vi "Check wether Click is in Plot Area.vi"(9 "Mouse Click Coordinates":T2, 11 "Plot Bounds":T1) -> (3 "Is in Plot Area?":bool)   [LabVIEW 2019]
uses:
  <vilib>/Utility/miscctls.llb/LVPoint32TypeDef.ctl
  <vilib>/Utility/miscctls.llb/LVRectTypeDef.ctl
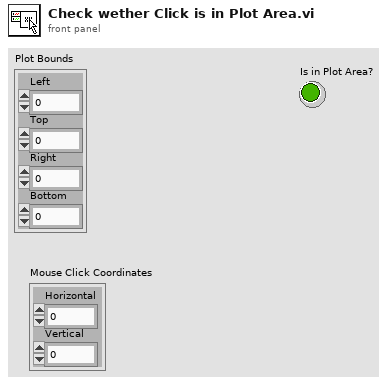
[diagram p1: front panel]
types:
  T1 = typedef "LVRectTypeDef.ctl" = cluster{"Left":i16, "Top":i16, "Right":i16, "Bottom":i16}
  T2 = typedef "LVPoint32TypeDef.ctl" = cluster{"Horizontal":i32, "Vertical":i32}
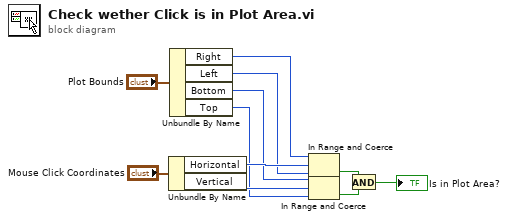
[diagram p0: block diagram]
diagram:
  n1 = Unbundle By Name("Mouse Click Coordinates") -> ("Horizontal"=w9:i32, "Vertical"=w6:i32)
  n2 = Unbundle By Name("Plot Bounds") -> ("Right"=w8:i16, "Left"=w7:i16, "Bottom"=w5:i16, "Top"=w4:i16)
  n3 = In Range and Coerce(upper limit=w8, x=w9, lower limit=w7) -> (In Range?=w3:bool)  [unwired: 1 out]
  n4 = In Range and Coerce(upper limit=w5, x=w6, lower limit=w4) -> (In Range?=w2:bool)  [unwired: 1 out]
  n5 = And(x=w3, y=w2) -> (x .and. y?=→"Is in Plot Area?":bool)
